vi "FPGA Main.vi"() -> ()   [LabVIEW 2020]
uses:
  <vilib>/Platform/TimedLoop/XDataNode/timing_clust.ctl
  <vilib>/Platform/TimedLoop/XDataNode/nitl_modes.ctl
  <vilib>/Platform/TimedLoop/XDataNode/wakeup.ctl
  <vilib>/rvi/Emulation/niFpgaSctlEmulationGetInTimedLoop.vi
  <vilib>/rvi/Emulation/niFpgaEmulationReportErrorSimple.vi
  <vilib>/rvi/Emulation/niFpgaGetClockAttributes.vi
  <vilib>/rvi/Emulation/niFpgaCriticalErrorInLSC.vi
  <vilib>/rvi/eio/common/nirviEmuTemplateMethod_errors.vi
  <vilib>/platform/TimedLoop/XDataNode/XDataNode.xnode
  <vilib>/eio/EIONode/EIONode.xnode
  <vilib>/Platform/TimedLoop/XDataNode/XDNodeRunTimeDep.lvlib
panel:
  out "Connector3":u32
  out "Connector2":u32
  out "Connector1":u32
  out "Connector0":u32
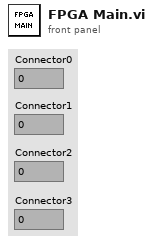
[diagram p1: front panel]
types:
  T1 = typedef "XDNodeRunTimeDep.lvlib/timing_clust.ctl" = cluster{"Expected End [f-1]":u64, "Actual End [f-1]":u64, "Finished Late? [f-1]":bool, "Expected End [i-1]":u64, "Actual End [i-1]":u64, "Finished Late? [i-1]":bool, "Expected Start [i]":u64, "Actual Start [i]":u64, "Expected Start [f]":u64, "Actual Start [f]":u64, "Source Name":string, "Structure Name":string, "Period":i64, "Deadline":i64, "Offset":i64, "Start":i64, "Priority":i32, "Timeout":i32, "Mode":T2, "Wakeup Reason":T3, "Error":errorcluster, "Source Type":string, "Secondary Source Type":string, "Global End Time":u64, "Global Start Time":u64, "Frame Duration":u64, "Iteration Duration":u64, "Assigned CPU":i32, "I/O Scan Engine Mode":u32}
  T2 = typedef "XDNodeRunTimeDep.lvlib/nitl_modes.ctl" = enum32{"No Change", "Process missed periods, maintain original phase", "Discard missed periods, maintain original phase", "Process missed periods, ignore original phase", "Discard missed periods, ignore original phase"}
  T3 = typedef "XDNodeRunTimeDep.lvlib/wakeup.ctl" = enum32{"Normal", "Aborted", "Asynchronous wakeup", "Timing source error", "Timed loop error", "Timeout"}
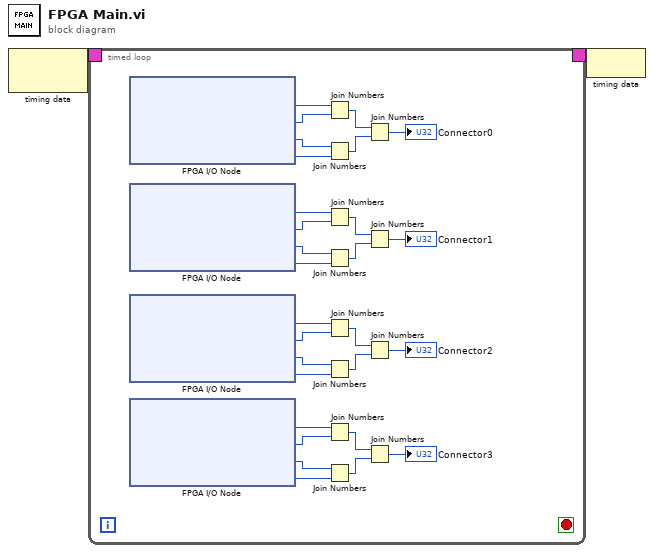
[diagram p0: block diagram]
diagram:
  n1 = node-c288() -> (w2:T1)  [unwired: 1 in]
  n2 = timed-loop {
    timing: w2 -> [_]
    timing-out: [_] -> w1
    stop <- _ stop-if-true
    n3 = xnode "FPGA I/O Node"() -> ("Connector0/DIOPORT3"=w29:u8, "Connector0/DIOPORT2"=w28:u8, "Connector0/DIOPORT1"=w27:u8, "Connector0/DIOPORT0"=w30:u8)  [unwired: 4 in, 4 out]
    n4 = xnode "FPGA I/O Node"() -> ("Connector1/DIOPORT3"=w18:u8, "Connector1/DIOPORT2"=w19:u8, "Connector1/DIOPORT1"=w20:u8, "Connector1/DIOPORT0"=w17:u8)  [unwired: 4 in, 4 out]
    n5 = xnode "FPGA I/O Node"() -> ("Connector2/DIOPORT3"=w15:u8, "Connector2/DIOPORT2"=w14:u8, "Connector2/DIOPORT1"=w13:u8, "Connector2/DIOPORT0"=w16:u8)  [unwired: 4 in, 4 out]
    n6 = xnode "FPGA I/O Node"() -> ("Connector3/DIOPORT3"=w4:u8, "Connector3/DIOPORT2"=w5:u8, "Connector3/DIOPORT1"=w6:u8, "Connector3/DIOPORT0"=w3:u8)  [unwired: 4 in, 4 out]
    n7 = Join Numbers(hi=w29, lo=w28) -> ((hi.lo)=w26:u16)
    n8 = Join Numbers(hi=w27, lo=w30) -> ((hi.lo)=w25:u16)
    n9 = Join Numbers(hi=w18, lo=w19) -> ((hi.lo)=w21:u16)
    n10 = Join Numbers(hi=w20, lo=w17) -> ((hi.lo)=w22:u16)
    n11 = Join Numbers(hi=w15, lo=w14) -> ((hi.lo)=w12:u16)
    n12 = Join Numbers(hi=w13, lo=w16) -> ((hi.lo)=w11:u16)
    n13 = Join Numbers(hi=w4, lo=w5) -> ((hi.lo)=w7:u16)
    n14 = Join Numbers(hi=w6, lo=w3) -> ((hi.lo)=w8:u16)
    n15 = Join Numbers(hi=w26, lo=w25) -> ((hi.lo)=→"Connector0":u32)
    n16 = Join Numbers(hi=w21, lo=w22) -> ((hi.lo)=→"Connector1":u32)
    n17 = Join Numbers(hi=w12, lo=w11) -> ((hi.lo)=→"Connector2":u32)
    n18 = Join Numbers(hi=w7, lo=w8) -> ((hi.lo)=→"Connector3":u32)
  }
  n19 = node-c288(w1) -> ()
